vi "PCO_GetRecorderSubmode.vi"(8 "error in (no error)":errorcluster {"code" format="%x"}, 11 "ph":u64) -> (0 "error out":errorcluster {"code" format="%x"}, 1 "wRecSubmode":u16(ring) items=["sequence", "ring buffer"], 2 "ErrorMessage":i32 format="%x", 3 "ph out":u64)   [LabVIEW 2019, in "SDK.lvlib" / "RecordingControl.lvlib"]
doc: "<b>Description:</b>\nThis function returns the current recorder submode of the camera. Recorder submode is only available if the storage mode is set to [recorder].\nRecorder submode is either [sequence] or [ring buffer].\n\n<b>Supported camera type:</b>\npco.dimax, pco.pixelfly usb, pco.ultraviolet, pco.1200, pco.1300, pco.1400, pco.1600, pco.2000, pco.4000\n\n<b>Descriptor dependency:</b>\ndwGeneralCapsDESC1: NO_RECORDER"
uses:
  RecordingControl.lvlib
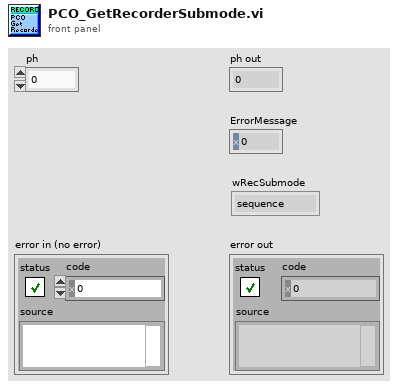
[diagram p1: front panel]
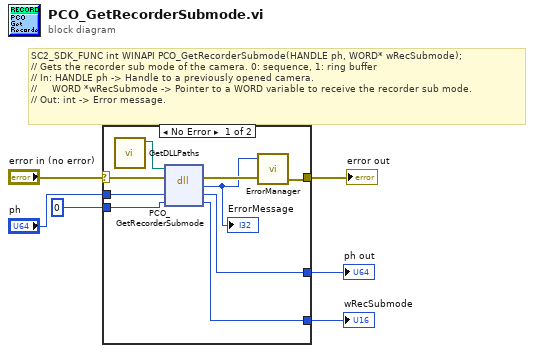
[diagram p0: block diagram]
diagram:
  # "SC2_SDK_FUNC int WINAPI PCO_GetRecorderSubmode(HANDLE ph, WORD* wRecSubmode);\n// Gets the recorder sub mode of the camera. 0: sequence, 1: ring buffer\n// In: HANDLE ph -> Handle to a previously opened camera.\n//     WORD *wRecSubmode -> Pointer to a WORD variable to receive the recorder sub mode.\n// Out: int -> Error message."
  n1 = case shown="No Error" "error in (no error)" {
    selector: "error in (no error)" -> [w11 w18]
    tunnel: "ph" -> [w15 w17]
    tunnel: [w14 w17] -> w5
    tunnel: u16 0 ("wRecSubmode") -> [w13 w16]
    tunnel: [w12 w16] -> w3
    tunnel: [w9 w18] -> w2
    frame No Error {
      n2 = call "GetDLLPaths.vi"() -> ("SC2_Cam_Path"=w7:path)  [unwired: 9 in, 2 out]
      n3 = dll-call lib="?" fn="PCO_GetRecorderSubmode"(path in=w7, error in=w11, "ph"=w15, "wRecSubmode"=w13) -> (error out=w10:errorcluster, "return type"=w8:i32, "ph"=w14:u64, "wRecSubmode"=w12:u16)  [unwired: 1 in, 1 out]
      "ErrorMessage" <- w8
      n4 = call "ErrorManager.vi"("error in (no error)"=w10, "error code"=w8) -> ("error out"=w9:errorcluster)  [unwired: 3 in]
    }
    frame Error {
    }
  }
  "ph out" <- w5
  "wRecSubmode" <- w3
  "error out" <- w2
